vi "Processamento_0405.vi"() -> ()   [LabVIEW 2017]
uses:
  <vilib>/userdefined/High Color/IMAQdx.ctl
  <vilib>/vision/driver/IMAQdx.llb/IMAQdx Acquisition Mode.ctl
  <vilib>/vision/driver/IMAQdx.llb/IMAQdx Buffer Number Mode.ctl
  <vilib>/vision/Measure.llb/Edge Options.ctl
  <vilib>/vision/Measure.llb/Edge Polarity.ctl
  <vilib>/vision/Measure.llb/Straight Edge Options.ctl
  <vilib>/vision/Measure.llb/Straight Edge Process.ctl
  <vilib>/vision/Classification.llb/IMAQ Classifier Read Options.ctl
  <vilib>/vision/driver/NI_Vision_Acquisition_Software.lvlib
  <vilib>/vision/NI_Vision_Development_Module.lvlib
  <resource>/objmgr/IMAQImage.rc
panel:
  in  "Período do histórico (s)":dbl min=0.0 step=0.1
  in  "Salvar dados":bool
  out "Table Control":string[][](table)
  in  "Histórico":path=path "C:/Users/Manufatura/Desktop/Jonas/CV/Histórico.txt"
  out "error out 3":errorcluster
  out "error out 2":errorcluster
  out "error out":errorcluster
  in  "Classificador de cor":path=path "C:/Users/Manufatura/Desktop/Jonas/CV/Classificador de cor.clf"
  out "Imagem Processada":T1(plugin-control)
  in  "Stop Button":bool
  out "Imagem Original":T1(plugin-control)
  in  "Câmera":T2="cam1"
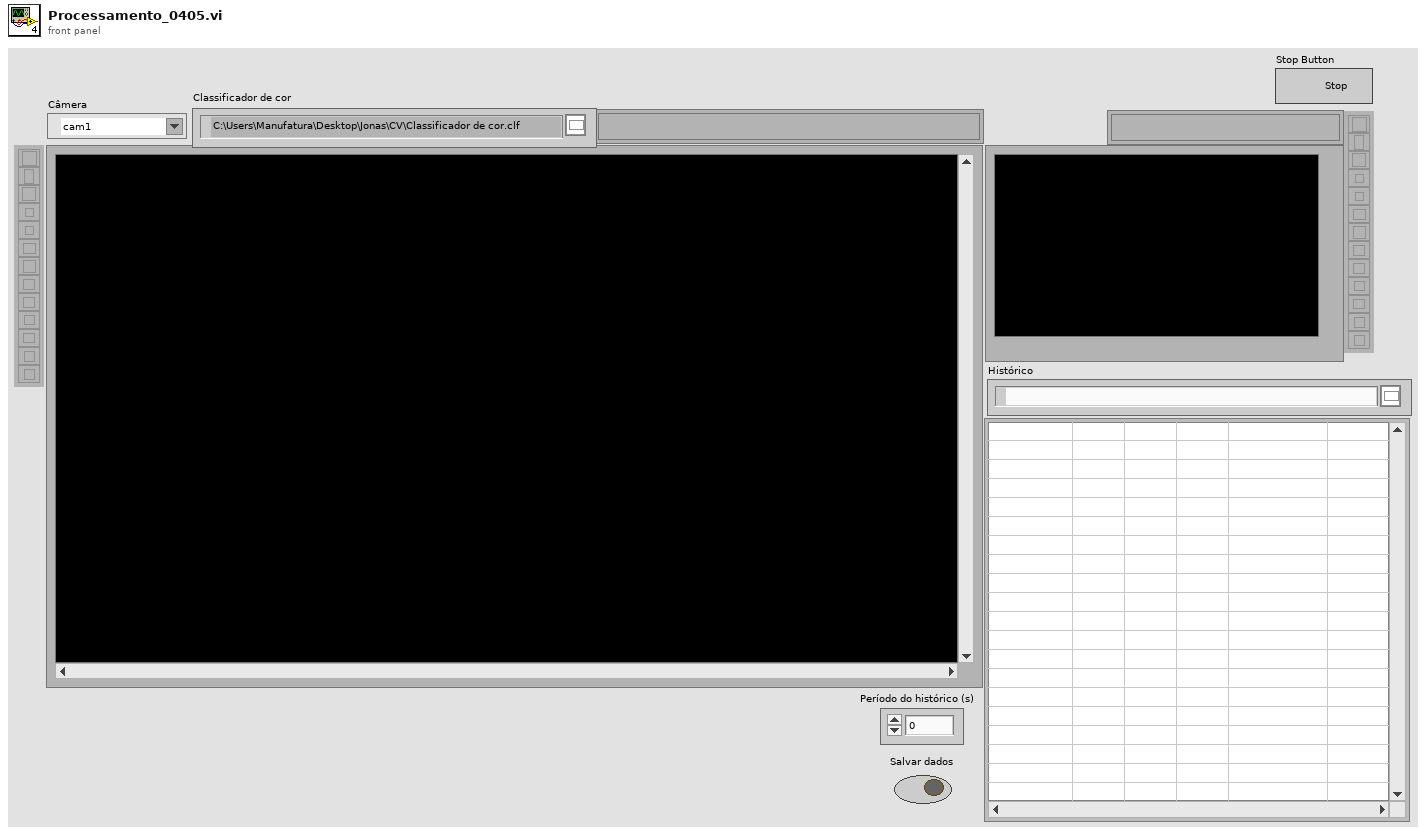
[diagram p1: front panel]
types:
  T1 = typedef "IMAQ Image.ctl" = refnum<image>
  T2 = typedef "IMAQdx.ctl" = refnum<k21>
  T3 = enum16{"open", "replace", "create", "open or create", "replace or create", "replace or create with confirmation"}
  T4 = typedef "Image Type" = u32
  T5 = typedef "NI_Vision_Acquisition_Software.lvlib/IMAQdx Acquisition Mode.ctl" = enum32{"One Shot", "Continuous"}
  T6 = cluster{"Objects":u16, "Threshold":i32, "Reject Border":bool, "Fill Holes":bool, "Min Object Size":bool, "Min Size":i32, "Max Object Size":bool, "Max Size":i32, "Show Search Area":bool, "Show Center":bool, "Show Bounding Box":bool}
  T7 = enum32{"AutoM", "Close", "Dilate", "Erode", "Gradient", "Gradient out", "Gradient in", "Hit miss", "Open", "PClose", "POpen", "Thick", "Thin"}
  T8 = typedef "Edge Options.ctl" = cluster{"Edge Polarity":T9, "Kernel Size":u32, "Width":u32, "Minimum Edge Strength":sgl, "Interpolation Type":enum32{"Zero Order", "Bilinear", "Quadratic", "Cubic", "Bilinear Fixed"}, "Data Processing Method":enum32{"Average", "Median"}}
  T9 = typedef "Edge Polarity.ctl" = u32
  T10 = cluster{"Search Direction":u32, "Edge Options":T8, "Show Search Area":bool, "Show Search Lines":bool, "Show Edges Found":bool, "Show Result":bool, "Search Area Color":u32, "Search Lines Color":u32, "Edge Locations Color":u32, "Result Color":u32, "Overlay Group Name":string}
  T11 = typedef "NI_Vision_Acquisition_Software.lvlib/IMAQdx Buffer Number Mode.ctl" = enum32{"Next", "Last", "Buffer Number", "Every", "Last New"}
  T12 = typedef "Straight Edge Options.ctl" = cluster{"Number of Lines":i32, "Type":T13, "Min. Score":dbl, "Max. Score":dbl, "Orientation":dbl, "Angle Range":dbl, "Angle Tolerance":dbl, "Step Size":u32, "Min. SNR (db)":dbl, "Min. Points (%)":dbl, "Hough Iterations":i32}
  T13 = typedef "Straight Edge Process.ctl" = enum32{"First Edge Rake", "Best Edge Rake", "Hough Edge Rake", "First Edge Projection", "Best Edge Projection"}
  T14 = cluster{"Desired Font (Application)":enum16{"User-specified Font", "Application Font", "System Font", "Dialog Font"}, "[User-specified Font]":cluster{"Font Name":string, "Size":i16, "Strikeout?":bool, "Italic?":bool, "Underline?":bool, "Outline?":bool, "Shadow?":bool, "Bold?":bool, "Rotation Angle":dbl}, "Horizontal Alignment":i16, "Vertical Alignment":i16}
  T15 = cluster{"Extraction Mode":u32, "Edge Threshold":i32, "Edge Filter Size":u32, "Min Length":i32, "Row Search Step Size":i32, "Col Search Step Size":i32, "Max Endpoint Gap":i32, "Closed":bool, "Subpixel":bool}
  T16 = cluster{"Rotation":bool, "Scale":bool, "Occlusion":bool, "Range Settings":cluster{"Match Constraints":u32, "Min":dbl, "Max":dbl}[]}
  T17 = cluster{"element":dbl, "y":i32, "x":i32, "element":dbl, "element":dbl}
  T18 = typedef "ROI Descriptor" = cluster{"Global Rectangle":i32[], "Contours":cluster{"ID":enum32{"External", "Internal"}, "Type":u32, "Coordinates":i32[]}[]}
  T19 = cluster{"Point1 (Pixels)":cluster{"X":sgl, "Y":sgl}, "Point2 (Pixels)":cluster{"X":sgl, "Y":sgl}, "Point1 (Real-World)":cluster{"X":sgl, "Y":sgl}, "Point2 (Real-World)":cluster{"X":sgl, "Y":sgl}, "Angle (Pixel)":dbl, "Angle (Real-World)":dbl, "Score":dbl, "Straightness":dbl, "Average SNR (db)":dbl, "Calibration Valid":bool}[]
  T20 = cluster{"Point1 (Pixels)":cluster{"X":sgl, "Y":sgl}, "Point2 (Pixels)":cluster{"X":sgl, "Y":sgl}, "Point1 (Real-World)":cluster{"X":sgl, "Y":sgl}, "Point2 (Real-World)":cluster{"X":sgl, "Y":sgl}, "Angle (Pixel)":dbl, "Angle (Real-World)":dbl, "Score":dbl, "Straightness":dbl, "Average SNR (db)":dbl, "Calibration Valid":bool}
  T21 = cluster{"element":dbl, sgl, "x":i32, sgl, "element":dbl}
  T22 = cluster{"Object Center":cluster{"X":sgl, "Y":sgl}, "Bounding Box":cluster{"X Left":i32, "Y Top":i32, "X Right":i32, "Y Bottom":i32}, "Area":sgl, "Orientation":sgl, "Aspect Ratio":sgl, "Nb Holes":i32}[]
  T23 = cluster{"X Left":i32, "Y Top":i32, "X Right":i32, "Y Bottom":i32}
  T24 = typedef "IMAQ Classifier Read Options.ctl" = i32
  T25 = typedef "IMAQ Classifier Session.ctl" = refnum<k1>
  T26 = cluster{i32, "Object Center":cluster{"X":sgl, "Y":sgl}, "Bounding Box":cluster{"X Left":i32, "Y Top":i32, "X Right":i32, "Y Bottom":i32}, "Angle (Pixel)":dbl, "Number of Matches Returned":i32}
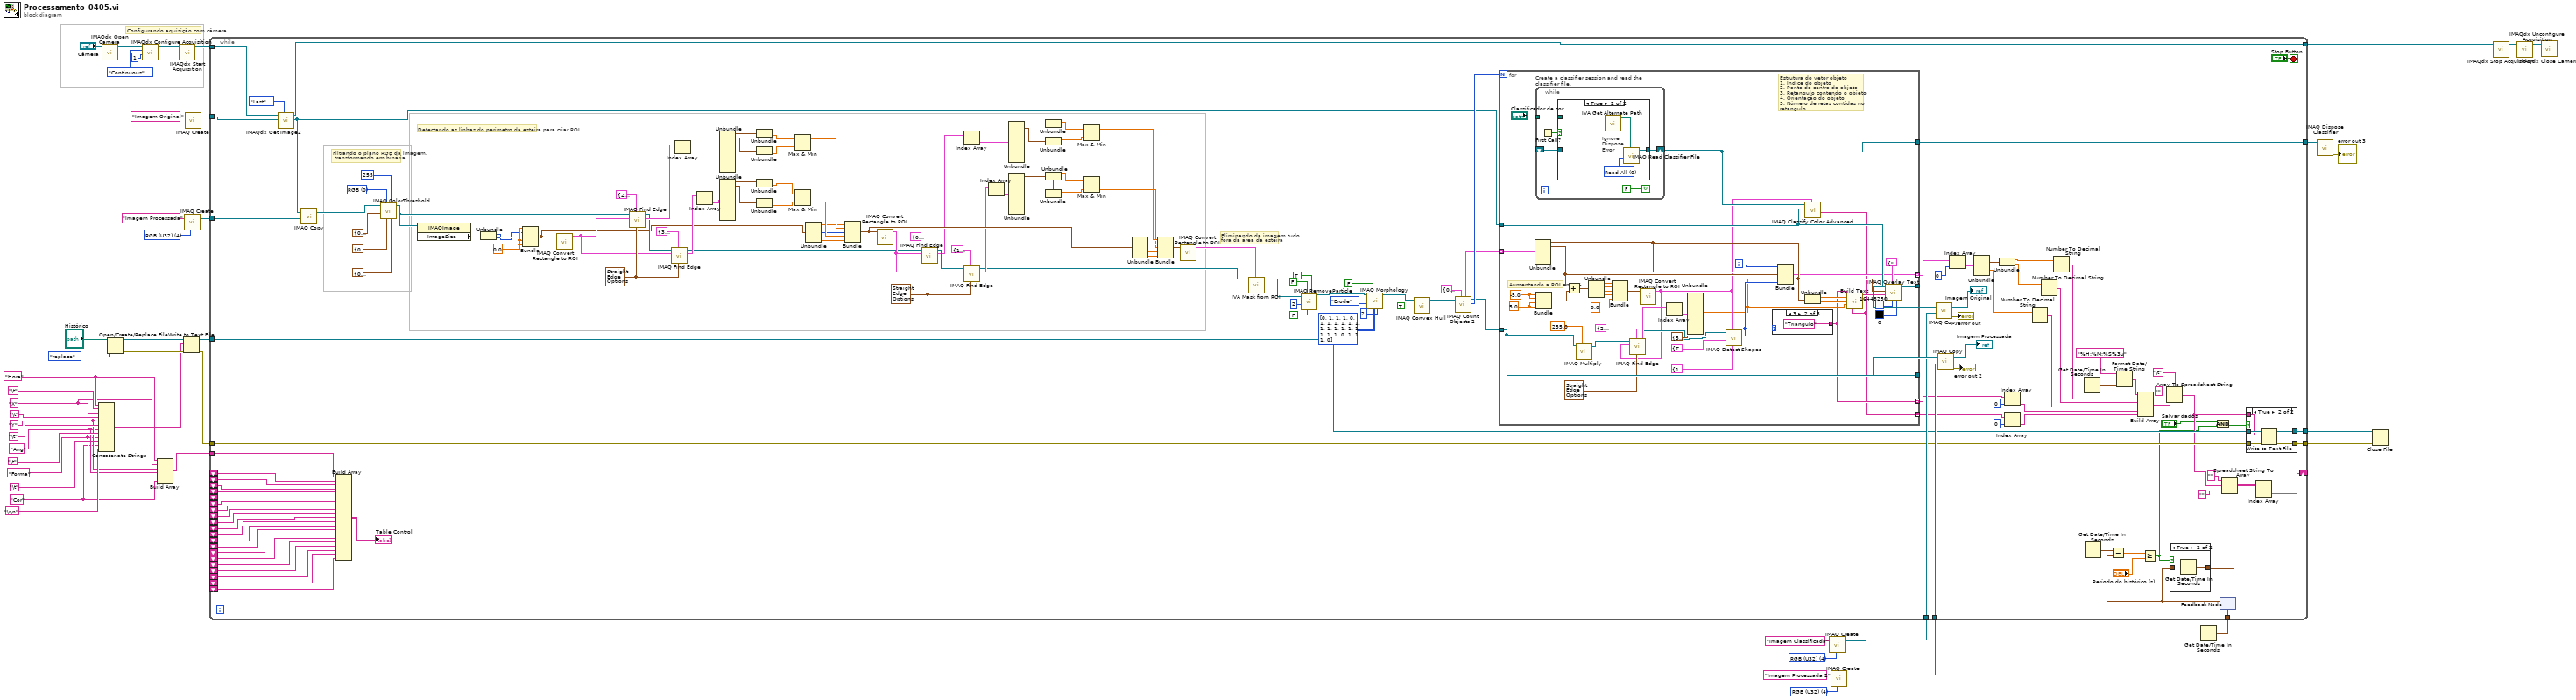
[diagram p0: block diagram]
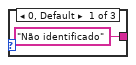
[diagram p4: hidden frame]
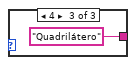
[diagram p5: hidden frame]
diagram:
  w8 = "Hora" ("string")
  w2 = "Cor" ("string")
  w4 = "Forma" ("string")
  w5 = "Ang" ("string")
  w6 = "Y" ("string")
  w7 = "X" ("string")
  w27 = T4 4 items=["Grayscale (U8)", "Grayscale (I16)", "Grayscale (SGL)", "Complex (CSG)", "RGB (U32)", "HSL (U32)", "RGB (U64)", "Grayscale (U16)"] ("Image Type")
  w30 = T4 4 items=["Grayscale (U8)", "Grayscale (I16)", "Grayscale (SGL)", "Complex (CSG)", "RGB (U32)", "HSL (U32)", "RGB (U64)", "Grayscale (U16)"] ("Image Type")
  w34 = T4 4 items=["Grayscale (U8)", "Grayscale (I16)", "Grayscale (SGL)", "Complex (CSG)", "RGB (U32)", "HSL (U32)", "RGB (U64)", "Grayscale (U16)"] ("Image Type")
  # "Configurando aquisição com câmera"
  n1 = Concatenate Strings(w8, "\t", w7, "\t", w6, "\t", w5, "\t", w4, "\t", w2, "\r\n") -> (w13:string)
  n2 = call <vilib>:"IMAQdx Open Camera.vi"("Session In"="Câmera") -> ("Session Out"=w45:T2)  [unwired: 9 in, 1 out]
  n3 = Open/Create/Replace File(file path (use dialog)="Histórico", operation (0:open)=T3."replace") -> (refnum out=w21:refnum<file>, error out=w20:errorcluster)  [unwired: 4 in, 1 out]
  n4 = call <vilib>:"IMAQdx Configure Acquisition.vi"("Number of Buffers"=u32 1, "Continuous?"=IMAQdx_Acquisition_Mode."Continuous", "Session In"=w45) -> ("Session Out"=w44:T2)  [unwired: 7 in, 1 out]
  n5 = Build Array(w8, w7, w6, w5, w4, w2) -> (w3:string[])
  n6 = call <vilib>:"IMAQdx Start Acquisition.vi"("Session In"=w44) -> ("Session Out"=w33:T2)  [unwired: 9 in, 1 out]
  n7 = Write to Text File(file (use dialog)=w21, text=w13, error in=w20) -> (refnum out=w11:refnum<file>, error out=w12:errorcluster)  [unwired: 1 in, 1 out]
  n8 = call "IMAQ Create"("Image Name"="Imagem Processada", "Image Type"=w34) -> ("New Image"=w35:T1)  [unwired: 3 in, 1 out]
  n9 = call "IMAQ Create"("Image Name"="Imagem Original") -> ("New Image"=w39:T1)  [unwired: 4 in, 1 out]
  n10 = call "IMAQ Create"("Image Name"="Imagem Classificada", "Image Type"=w27) -> ("New Image"=w26:T1)  [unwired: 3 in, 1 out]
  n11 = call "IMAQ Create"("Image Name"="Imagem Processada 2", "Image Type"=w30) -> ("New Image"=w29:T1)  [unwired: 3 in, 1 out]
  n12 = Get Date/Time In Seconds() -> (seconds since 1Jan1904=w1:timestamp)
  n13 = while {
    tunnel: w39 -> [w201]
    tunnel: w35 -> [w198]
    tunnel: w33 -> [w122]
    tunnel: [w121] -> w32
    tunnel: w29 -> [w115]
    tunnel: w26 -> [w112]
    tunnel: [w110] -> w25
    tunnel: w12 -> [w86]
    tunnel: w11 -> [w85]
    tunnel: [w84] -> w10
    tunnel: [w83] -> w9
    shift-right: [w61] -> _
    shift-left: _ -> [w82]
    shift-left: _ -> [w81]
    shift-left: _ -> [w80]
    shift-left: _ -> [w79]
    shift-left: _ -> [w78]
    shift-left: _ -> [w77]
    shift-left: _ -> [w76]
    shift-left: _ -> [w75]
    shift-left: _ -> [w74]
    shift-left: _ -> [w73]
    shift-left: _ -> [w72]
    shift-left: _ -> [w71]
    shift-left: _ -> [w70]
    shift-left: _ -> [w69]
    shift-left: _ -> [w68]
    shift-left: _ -> [w67]
    shift-left: _ -> [w66]
    shift-left: _ -> [w65]
    shift-left: _ -> [w64]
    shift-left: _ -> [w63]
    tunnel: w3 -> [w59]
    tunnel: w1 -> [w52]
    stop <- "Stop Button" stop-if-true
    w159 = T12 {"Number of Lines"=1, "Type"=enum."First Edge Rake", "Min. Score"=10.0, "Max. Score"=1000.0, "Orientation"=0.0, "Angle Range"=45.0, "Angle Tolerance"=1.0, "Step Size"=32, "Min. SNR (db)"=0.0, "Min. Points (%)"=25.0, "Hough Iterations"=5} ("Fit Options")
    w184 = T12 {"Number of Lines"=1, "Type"=enum."First Edge Rake", "Min. Score"=10.0, "Max. Score"=1000.0, "Orientation"=0.0, "Angle Range"=45.0, "Angle Tolerance"=1.0, "Step Size"=32, "Min. SNR (db)"=0.0, "Min. Points (%)"=25.0, "Hough Iterations"=5} ("Fit Options")
    w190 = 0.0 ("element")
    w193 = u16 0 items=["RGB", "HSL", "HSV", "HSI"] ("Color Mode")
    # "Eliminando da imagem tudo\nfora da área da esteira"
    # "Detectando as linhas do perimetro da esteira para criar ROI"
    # "Filtrando o plano RGB da imagem,\n transformando em binária"
    n14 = call <vilib>:"IMAQdx Get Image2.vi"("Buffer Number Mode (Next)"=IMAQdx_Buffer_Number_Mode."Last", "Image In"=w201, "Session In"=w122) -> ("Image Out"=w118:T1, "Session Out"=w121:T2)  [unwired: 5 in, 2 out]
    n15 = call "IMAQ Copy"("Image Dst"=w198, "Image Src"=w118) -> ("Image Dst Out"=w192:T1)  [unwired: 4 in, 1 out]
    n16 = Build Array(w59, w82, w81, w80, w79, w78, w77, w76, w75, w74, w73, w72, w71, w70, w69, w68, w67, w66, w65, w64, w63) -> (→"Table Control":string[][])
    n17 = call "IMAQ ColorThreshold"("Blue or Luma or Val or Inten Range"=cluster{"Lower value":i32, "Upper value":i32} {"Lower value"=0, "Upper value"=170}, "Replace Value"=255, "Green or Sat Range"=cluster{"Lower value":i32, "Upper value":i32} {"Lower value"=0, "Upper value"=255}, "Color Mode"=w193, "Red or Hue Range"=cluster{"Lower value":i32, "Upper value":i32} {"Lower value"=0, "Upper value"=255}, "Image Src"=w192) -> ("Image Dst Out"=w188:T1)  [unwired: 2 in, 3 out]
    n18 = property class="IMAQImage"(reference=w188) -> ("ImageSize"=w191:cluster{"x":i32, "y":i32})  [unwired: 1 in, 2 out]
    n19 = Unbundle(w191) -> ("x"=w187:i32, "y"=w186:i32)
    n20 = Bundle("element"=w190, "y"=w186, "x"=w187, "element"=w190, "element"=w190) -> (w157:T17)  [unwired: 1 in]
    n21 = call "IMAQ Convert Rectangle to ROI"("Rectangle"=w157) -> ("ROI Descriptor"=w183:T18)  [unwired: 8 in, 1 out]
    n22 = call "IMAQ Find Edge"("Line Fit Options"=w184, "Options"=T10 {"Search Direction"=2, "Edge Options"={"Edge Polarity"=2, "Kernel Size"=3, "Width"=1, "Minimum Edge Strength"=80.0, "Interpolation Type"=enum."Bilinear Fixed", "Data Processing Method"=enum."Average"}, "Show Search Area"=FALSE, "Show Search Lines"=FALSE, "Show Edges Found"=FALSE, "Show Result"=FALSE, "Search Area Color"=65280, "Search Lines Color"=255, "Edge Locations Color"=16776960, "Result Color"=16711680, "Overlay Group Name"=""}, "ROI Descriptor"=w183, "Image"=w188) -> ("Straight Edges"=w185:T19, "Image Out"=w182:T1)  [unwired: 2 in, 4 out]
    n23 = call "IMAQ Find Edge"("Line Fit Options"=w184, "Options"=T10 {"Search Direction"=3, "Edge Options"={"Edge Polarity"=2, "Kernel Size"=3, "Width"=1, "Minimum Edge Strength"=80.0, "Interpolation Type"=enum."Bilinear Fixed", "Data Processing Method"=enum."Average"}, "Show Search Area"=FALSE, "Show Search Lines"=FALSE, "Show Edges Found"=FALSE, "Show Result"=FALSE, "Search Area Color"=65280, "Search Lines Color"=255, "Edge Locations Color"=16776960, "Result Color"=16711680, "Overlay Group Name"=""}, "ROI Descriptor"=w183, "Image"=w182) -> ("Straight Edges"=w180:T19, "Image Out"=w160:T1)  [unwired: 2 in, 4 out]
    n24 = Index Array(array=w185) -> (element=w179:T20)  [unwired: 1 in]
    n25 = Index Array(array=w180) -> (element=w178:T20)  [unwired: 1 in]
    n26 = Unbundle(w179) -> ("Point1 (Pixels)"=w177:cluster{"X":sgl, "Y":sgl}, "Point2 (Pixels)"=w176:cluster{"X":sgl, "Y":sgl})  [unwired: 8 out]
    n27 = Unbundle(w178) -> ("Point1 (Pixels)"=w175:cluster{"X":sgl, "Y":sgl}, "Point2 (Pixels)"=w174:cluster{"X":sgl, "Y":sgl})  [unwired: 8 out]
    n28 = Unbundle(w177) -> ("Y"=w173:sgl)  [unwired: 1 out]
    n29 = Unbundle(w176) -> ("Y"=w172:sgl)  [unwired: 1 out]
    n30 = Unbundle(w175) -> ("Y"=w171:sgl)  [unwired: 1 out]
    n31 = Unbundle(w174) -> ("Y"=w170:sgl)  [unwired: 1 out]
    n32 = Max & Min(x=w173, y=w172) -> (max(x,y)=w169:sgl)  [unwired: 1 out]
    n33 = Max & Min(x=w171, y=w170) -> (min(x,y)=w168:sgl)  [unwired: 1 out]
    n34 = Unbundle(w157) -> ("element"=w166:dbl, "x"=w167:i32, "element"=w165:dbl)  [unwired: 2 out]
    n35 = Bundle("element"=w166, w169, "x"=w167, w168, "element"=w165) -> (w155:T21)  [unwired: 1 in]
    n36 = call "IMAQ Convert Rectangle to ROI"("Rectangle"=w155) -> ("ROI Descriptor"=w162:T18)  [unwired: 8 in, 1 out]
    n37 = call "IMAQ Find Edge"("Line Fit Options"=w159, "Options"=T10 {"Search Direction"=0, "Edge Options"={"Edge Polarity"=2, "Kernel Size"=3, "Width"=1, "Minimum Edge Strength"=80.0, "Interpolation Type"=enum."Bilinear Fixed", "Data Processing Method"=enum."Average"}, "Show Search Area"=FALSE, "Show Search Lines"=FALSE, "Show Edges Found"=FALSE, "Show Result"=FALSE, "Search Area Color"=65280, "Search Lines Color"=255, "Edge Locations Color"=16776960, "Result Color"=16711680, "Overlay Group Name"=""}, "ROI Descriptor"=w162, "Image"=w160) -> ("Straight Edges"=w146:T19, "Image Out"=w161:T1)  [unwired: 2 in, 4 out]
    n38 = Index Array(array=w146) -> (element=w150:T20)  [unwired: 1 in]
    n39 = call "IMAQ Find Edge"("Line Fit Options"=w159, "Options"=T10 {"Search Direction"=1, "Edge Options"={"Edge Polarity"=2, "Kernel Size"=3, "Width"=1, "Minimum Edge Strength"=80.0, "Interpolation Type"=enum."Bilinear Fixed", "Data Processing Method"=enum."Average"}, "Show Search Area"=FALSE, "Show Search Lines"=FALSE, "Show Edges Found"=FALSE, "Show Result"=FALSE, "Search Area Color"=65280, "Search Lines Color"=255, "Edge Locations Color"=16776960, "Result Color"=16711680, "Overlay Group Name"=""}, "ROI Descriptor"=w162, "Image"=w161) -> ("Straight Edges"=w145:T19, "Image Out"=w137:T1)  [unwired: 2 in, 4 out]
    n40 = Index Array(array=w145) -> (element=w149:T20)  [unwired: 1 in]
    n41 = Unbundle(w150) -> ("Point1 (Pixels)"=w151:cluster{"X":sgl, "Y":sgl}, "Point2 (Pixels)"=w152:cluster{"X":sgl, "Y":sgl})  [unwired: 8 out]
    n42 = Unbundle(w149) -> ("Point1 (Pixels)"=w148:cluster{"X":sgl, "Y":sgl}, "Point2 (Pixels)"=w147:cluster{"X":sgl, "Y":sgl})  [unwired: 8 out]
    n43 = Unbundle(w151) -> ("X"=w142:sgl)  [unwired: 1 out]
    n44 = Unbundle(w152) -> ("X"=w141:sgl)  [unwired: 1 out]
    n45 = Unbundle(w148) -> ("X"=w140:sgl)  [unwired: 1 out]
    n46 = Unbundle(w147) -> ("X"=w139:sgl)  [unwired: 1 out]
    n47 = Max & Min(x=w142, y=w141) -> (max(x,y)=w144:sgl)  [unwired: 1 out]
    n48 = Max & Min(x=w140, y=w139) -> (min(x,y)=w143:sgl)  [unwired: 1 out]
    n49 = Unbundle(w155) -> (w154:sgl, w153:sgl, "element"=w156:dbl)  [unwired: 2 out]
    n50 = Bundle(w144, w154, w143, w153, "element"=w156) -> (w158:cluster{sgl, sgl, sgl, sgl, "element":dbl})  [unwired: 1 in]
    n51 = call "IMAQ Convert Rectangle to ROI"("Rectangle"=w158) -> ("ROI Descriptor"=w138:T18)  [unwired: 8 in, 1 out]
    n52 = call <vilib>:"IVA Mask from ROI.vi"("ROI Descriptor"=w138, "Image Src"=w137) -> ("Image Out"=w132:T1)  [unwired: 3 in, 6 out]
    n53 = call "IMAQ RemoveParticle"("Connectivity 4/8 (8)"=TRUE, "Low Pass/High Pass (Low)"=FALSE, "Square/Hexa (Square)"=FALSE, "Number of Erosion"=2, "Image Src"=w132) -> ("Image Dst Out"=w127:T1)  [unwired: 2 in, 4 out]
    n54 = call "IMAQ Morphology"("Number of iterations (1)"=2, "Structuring Element"=i32[][] [[0, 1, 1, 1, 0], [1, 1, 1, 1, 1], [1, 1, 1, 1, 1], [1, 1, 1, 1, 1], [0, 1, 1, 1, 0]], "Square/Hexa (Square)"=FALSE, "Operation"=T7."Erode", "Image Src"=w127) -> ("Image Dst Out"=w125:T1)  [unwired: 2 in, 4 out]
    n55 = call "IMAQ Convex Hull"("Connectivity 4/8 (8)"=TRUE, "Image Src"=w125) -> ("Image Dst Out"=w124:T1)  [unwired: 2 in, 7 out]
    n56 = call "IMAQ Count Objects 2"("Settings"=T6 {"Objects"=0, "Threshold"=1, "Reject Border"=FALSE, "Fill Holes"=FALSE, "Min Object Size"=TRUE, "Min Size"=400, "Max Object Size"=FALSE, "Max Size"=100, "Show Search Area"=FALSE, "Show Center"=FALSE, "Show Bounding Box"=FALSE}, "Image"=w124) -> ("Number of Objects"=w120:i32, "Image Out"=w117:T1, "Objects"=w119:T22)  [unwired: 5 in, 2 out]
    n57 = for {
      N: w120 -> [_]
      tunnel: w119 -> [w248] mode=indexing
      tunnel: w118 -> [w229]
      tunnel: w117 -> [w224]
      tunnel: [w224] -> w116
      tunnel: [w231] -> w113
      tunnel: [w227] -> w110
      tunnel: [w226] -> w105 mode=indexing
      tunnel: [w212] -> w92 mode=indexing
      tunnel: [w211] -> w89 mode=indexing
      i -> [w237]
      w247 = -5.0
      w246 = 5.0
      # "Estrutura do vetor objeto\n1. Indice do objeto\n2. Ponto do centro do objeto\n3. Retangulo contendo o objeto\n4. Orientação do objeto\n5. Número de retas contidas no retangulo"
      # "Aumentando a ROI em 5%"
      n58 = Unbundle(w248) -> ("Object Center"=w234:cluster{"X":sgl, "Y":sgl}, "Bounding Box"=w228:T23)  [unwired: 4 out]
      n59 = while "Create a classifier session and read the classifier file." {
        shift-right: [w259] -> w227
        shift-left: _ -> [w255]
        tunnel: "Classificador de cor" -> [w257]
        stop <- FALSE continue-if-true
        n60 = First Call?() -> (First Call?: T/F=w256:bool)
        n61 = case shown="True" w256 {
          tunnel: [w260 w263] -> w259
          tunnel: w257 -> [_ w262]
          tunnel: w255 -> [w260 _]
          frame False {
          }
          frame True {
            w264 = T24 0 items=["Read All", "Add Samples, Do Not Change Options", "Read Options, Do Not Add Samples"] ("Read Options")
            # "Ignore Dispose Error"
            n62 = call <vilib>:"IVA Get Alternate Path.vi"("Path In"=w262) -> ("Path Out"=w261:path)  [unwired: 10 out]
            n63 = call "IMAQ Read Classifier File"("File Path"=w261, "Read Options"=w264) -> ("Classifier Session"=w263:T25)  [unwired: 2 in, 7 out]
          }
        }
      }
      n64 = Bundle(w247, w247, w246, w246) -> (w245:cluster{dbl, dbl, dbl, dbl})  [unwired: 1 in]
      n65 = Add(x=w228, y=w245) -> (x+y=w244:cluster{dbl, dbl, dbl, dbl})
      n66 = call "IMAQ Multiply"("Image Src A"=w224, "Constant"=255.0) -> ("Image Dst Out"=w222:T1)  [unwired: 5 in, 1 out]
      n67 = Unbundle(w244) -> (w243:dbl, w242:dbl, w241:dbl, w240:dbl)
      n68 = Bundle(w243, w242, w241, w240, 0.0) -> (w238:cluster{dbl, dbl, dbl, dbl, dbl})  [unwired: 1 in]
      n69 = call "IMAQ Convert Rectangle to ROI"("Rectangle"=w238) -> ("ROI Descriptor"=w217:T18)  [unwired: 8 in, 1 out]
      n70 = call "IMAQ Find Edge"("Line Fit Options"=T12 {"Number of Lines"=1, "Type"=enum."First Edge Rake", "Min. Score"=10.0, "Max. Score"=1000.0, "Orientation"=0.0, "Angle Range"=180.0, "Angle Tolerance"=1.0, "Step Size"=32, "Min. SNR (db)"=0.0, "Min. Points (%)"=25.0, "Hough Iterations"=5} ("Fit Options"), "Options"=T10 {"Search Direction"=2, "Edge Options"={"Edge Polarity"=2, "Kernel Size"=3, "Width"=1, "Minimum Edge Strength"=80.0, "Interpolation Type"=enum."Bilinear Fixed", "Data Processing Method"=enum."Average"}, "Show Search Area"=TRUE, "Show Search Lines"=TRUE, "Show Edges Found"=TRUE, "Show Result"=TRUE, "Search Area Color"=65280, "Search Lines Color"=255, "Edge Locations Color"=16776960, "Result Color"=16711680, "Overlay Group Name"=""}, "ROI Descriptor"=w217, "Image"=w222) -> ("Straight Edges"=w219:T19, "Image Out"=w218:T1)  [unwired: 4 in, 2 out]
      n71 = Index Array(array=w219) -> (element=w225:T20)  [unwired: 1 in]
      n72 = Unbundle(w225) -> ("Angle (Pixel)"=w215:dbl)  [unwired: 9 out]
      n73 = call-poly "IMAQ Detect Shapes"("Curve Parameters"=T15 {"Extraction Mode"=1, "Edge Threshold"=1, "Edge Filter Size"=1, "Min Length"=50, "Row Search Step Size"=15, "Col Search Step Size"=15, "Max Endpoint Gap"=10, "Closed"=FALSE, "Subpixel"=FALSE}, "ROI Descriptor"=w217, "Match Options"=T16 {"Rotation"=TRUE, "Scale"=FALSE, "Occlusion"=FALSE, "Range Settings"=[{"Match Constraints"=0, "Min"=0.0, "Max"=360.0}]}, "Line Descriptor"=cluster{"Min Length":dbl, "Max Length":dbl} {"Min Length"=50.0, "Max Length"=500.0}, "Image"=w218) -> ("Number of Matches Returned"=w216:i32)  [unwired: 4 in, 2 out]
      n74 = case shown="3" w216 {
        tunnel: ["Não identificado" "Triângulo" "Quadrilátero"] -> w212
        frame 0, Default {
        }
        frame 3 {
        }
        frame 4 {
        }
      }
      n75 = Bundle(w237, "Object Center"=w234, "Bounding Box"=w228, "Angle (Pixel)"=w215, "Number of Matches Returned"=w216) -> (w226:T26)  [unwired: 1 in]
      n76 = Unbundle(w234) -> ("X"=w213:sgl, "Y"=w214:sgl)
      n77 = call "IMAQ Classify Color Advanced"("ROI Descriptor"=w217, "Image"=w229, "Classifier Session"=w227) -> ("Class"=w211:string)  [unwired: 1 in, 7 out]
      n78 = call "Build Text"("forma"=w212, "x"=w213, "y"=w214, "orientação"=w215, "cor"=w211) -> ("Result"=w235:string)  [unwired: 9 in, 1 out]
      n79 = call "IMAQ Overlay Text"("BG Color (Transparent)"=u32 0, "Text Color (black)"=u32 16448250, "Font, Size & Style"=T14 {"Desired Font (Application)"=enum."Application Font", "[User-specified Font]"={"Font Name"="", "Size"=12, "Strikeout?"=FALSE, "Italic?"=FALSE, "Underline?"=FALSE, "Outline?"=FALSE, "Shadow?"=FALSE, "Bold?"=TRUE, "Rotation Angle"=0.0}, "Horizontal Alignment"=1, "Vertical Alignment"=2}, "String"=w235, "Origin"=w234, "Image"=w229) -> ("Image Out"=w231:T1)  [unwired: 4 in, 1 out]
    }
    n80 = call "IMAQ Copy"("Image Dst"=w112, "Image Src"=w113) -> ("error out"=→"error out":errorcluster, "Image Dst Out"=→"Imagem Original":T1)  [unwired: 4 in]
    n81 = call "IMAQ Copy"("Image Dst"=w115, "Image Src"=w116) -> ("error out"=→"error out 2":errorcluster, "Image Dst Out"=→"Imagem Processada":T1)  [unwired: 4 in]
    n82 = Index Array(array=w105, index=0) -> (element=w103:T26)
    n83 = Unbundle(w103) -> ("Object Center"=w102:cluster{"X":sgl, "Y":sgl}, "Angle (Pixel)"=w97:dbl)  [unwired: 3 out]
    n84 = Unbundle(w102) -> ("X"=w101:sgl, "Y"=w99:sgl)
    n85 = Index Array(array=w92, index=0) -> (element=w91:string)
    n86 = Index Array(array=w89, index=0) -> (element=w88:string)
    n87 = Number To Decimal String(number=w97) -> (decimal integer string=w96:string)  [unwired: 1 in]
    n88 = Number To Decimal String(number=w99) -> (decimal integer string=w98:string)  [unwired: 1 in]
    n89 = Number To Decimal String(number=w101) -> (decimal integer string=w100:string)  [unwired: 1 in]
    n90 = Get Date/Time In Seconds() -> (seconds since 1Jan1904=w58:timestamp)
    n91 = Get Date/Time In Seconds() -> (seconds since 1Jan1904=w51:timestamp)
    n92 = Format Date/Time String(time format string (%c)="%H:%M:%S%3u", seconds (now)=w58) -> (date/time string=w106:string)  [unwired: 1 in]
    n93 = Build Array(w106, w100, w98, w96, w91, w88) -> (w107:string[])
    n94 = Array To Spreadsheet String(delimiter (Tab)="\t", array=w107, 3:"" ("format string")) -> (spreadsheet string=w62:string)
    n95 = feedback #1(w52) -> (w49:timestamp)
    n96 = Subtract(x=w51, y=w49) -> (x-y=w50:dbl)
    n97 = Greater Or Equal?(x=w50, y="Período do histórico (s)") -> (x >= y?=w47:bool)
    n98 = case shown="True" w47 {
      tunnel: [w202 w203] -> w53
      tunnel: w49 -> [w202 _]
      frame False {
      }
      frame True {
        n99 = Get Date/Time In Seconds() -> (seconds since 1Jan1904=w203:timestamp)
      }
    }
    n100 = And(x="Salvar dados", y=w47) -> (x .and. y?=w46:bool)
    n101 = feedback-in #1(w53) -> ()
    n102 = Spreadsheet String To Array(format string="", spreadsheet string=w62, array type (2D Dbl)="" ("format string")) -> (array=w55:string[][])  [unwired: 1 in]
    n103 = case shown="True" w46 {
      tunnel: w86 -> [w204 w210]
      tunnel: w85 -> [w205 w209]
      tunnel: [w204 w208] -> w84
      tunnel: [w205 w207] -> w83
      tunnel: w62 -> [_ w206]
      frame False {
      }
      frame True {
        n104 = Write to Text File(file (use dialog)=w209, text=w206, error in=w210) -> (refnum out=w207:refnum<file>, error out=w208:errorcluster)  [unwired: 1 in, 1 out]
      }
    }
    n105 = Index Array(array=w55) -> (element=w61:string[])  [unwired: 2 in]
  }
  n106 = call "IMAQ Dispose Classifier"("Classifier Session"=w25) -> ("error out"=→"error out 3":errorcluster)  [unwired: 1 in, 9 out]
  n107 = Close File(refnum=w9, error in=w10) -> ()  [unwired: 2 out]
  n108 = call <vilib>:"IMAQdx Stop Acquisition.vi"("Session In"=w32) -> ("Session Out"=w43:T2)  [unwired: 9 in, 1 out]
  n109 = call <vilib>:"IMAQdx Unconfigure Acquisition.vi"("Session In"=w43) -> ("Session Out"=w42:T2)  [unwired: 9 in, 1 out]
  n110 = call <vilib>:"IMAQdx Close Camera.vi"("Session In"=w42) -> ()  [unwired: 10 in, 1 out]
